vi "Example Write File.vi"() -> ()   [LabVIEW 2013]
uses:
  C:/tf/play/labview/Tinkerforge.dll
  Tinkerforge.dll
panel:
  out "transferred (byte)":i32
  in  "local path":path=path "C:/foobar.txt"
  in  "remote path":string="/home/tf/foobar.txt"
  in  "uid":string="XXYYZZ"
  in  "port":i32=4223
  in  "host":string="localhost"
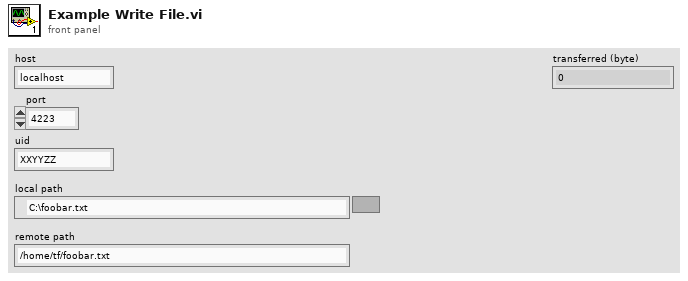
[diagram p1: front panel]
types:
  T1 = enum16{"open", "replace", "create", "open or create", "replace or create", "replace or create with confirmation"}
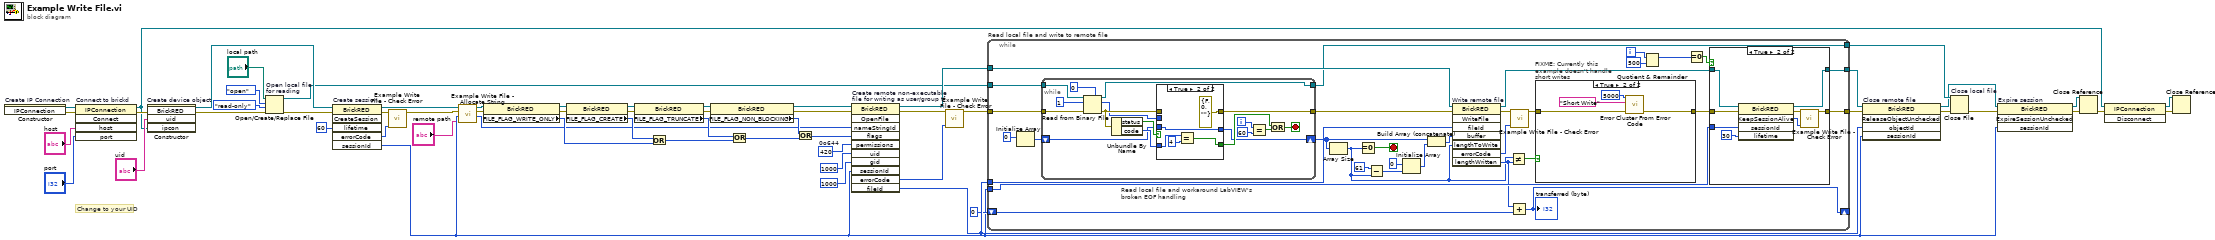
[diagram p0: block diagram]
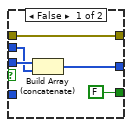
[diagram p2: hidden frame]
diagram:
  w41 = 420  # 0o644
  # "Change to your UID"
  n1 = constructor on="Create IP Connection" class="IPConnection"() -> (reference out=w59:refnum<k24>, error out=w49:errorcluster)  [unwired: 3 in, 1 out]
  n2 = invoke on="Connect to brickd" class="IPConnection" method="Connect"(reference=w59, error in=w49, "host"="host", "port"="port") -> (reference out=w51:refnum<k24>, error out=w55:errorcluster)  [unwired: 1 in, 3 out]
  n3 = constructor on="Create device object" class="BrickRED"(error in=w55, "uid"="uid", "ipcon"=w51) -> (reference out=w54:refnum<k24>, error out=w25:errorcluster)  [unwired: 2 in, 3 out]
  n4 = Open/Create/Replace File "Open local file\nfor reading"(file path (use dialog)="local path", error in=w25, operation (0:open)=T1."open", access (0:read/write)=enum16{"read/write", "read-only", "write-only"}."read-only") -> (refnum out=w35:refnum<file>, error out=w24:errorcluster)  [unwired: 2 in, 1 out]
  n5 = invoke on="Create session" class="BrickRED" method="CreateSession"(reference=w54, error in=w24, "lifetime"=i64 60) -> (reference out=w6:refnum<k24>, error out=w47:errorcluster, "errorCode"=w46:u8, "sessionId"=w2:i32)  [unwired: 3 in, 2 out]
  n6 = call "Example Write File - Check Error.vi"("error code"=w46, "error in"=w47) -> ("error out"=w7:errorcluster)  [unwired: 9 in]
  n7 = call "Example Write File - Allocate String.vi"("buffer"="remote path", "session id"=w2, "error in"=w7, "reference in"=w6) -> ("string id"=w3:i32, "error out"=w4:errorcluster, "reference out"=w5:refnum<k24>)  [unwired: 5 in]
  n8 = property class="BrickRED"(reference=w5, error in=w4) -> (reference out=w22:refnum<k24>, error out=w23:errorcluster, "FILE_FLAG_WRITE_ONLY"=w20:i64)
  n9 = property class="BrickRED"(reference=w22, error in=w23) -> (reference out=w18:refnum<k24>, error out=w15:errorcluster, "FILE_FLAG_CREATE"=w21:i64)
  n10 = property class="BrickRED"(reference=w18, error in=w15) -> (reference out=w17:refnum<k24>, error out=w16:errorcluster, "FILE_FLAG_TRUNCATE"=w14:i64)
  n11 = Or(x=w21, y=w20) -> (x .or. y?=w19:i64)
  n12 = property class="BrickRED"(reference=w17, error in=w16) -> (reference out=w39:refnum<k24>, error out=w40:errorcluster, "FILE_FLAG_NON_BLOCKING"=w11:i64)
  n13 = Or(x=w14, y=w19) -> (x .or. y?=w12:i64)
  n14 = Or(x=w11, y=w12) -> (x .or. y?=w13:i64)
  n15 = invoke on="Create remote non-executable\nfile for writing as user/group tf" class="BrickRED" method="OpenFile"(reference=w39, error in=w40, "nameStringId"=w3, "flags"=w13, "permissions"=w41, "uid"=i64 1000, "gid"=i64 1000, "sessionId"=w2) -> (reference out=w36:refnum<k24>, error out=w44:errorcluster, "errorCode"=w45:u8, "fileId"=w33:i32)  [unwired: 3 in, 7 out]
  n16 = call "Example Write File - Check Error.vi"("error code"=w45, "error in"=w44) -> ("error out"=w26:errorcluster)  [unwired: 9 in]
  n17 = while "Read local file and write to remote file" {
    tunnel: w26 -> [w73]
    tunnel: [w82] -> w10
    tunnel: w36 -> [w91]
    tunnel: [w83] -> w32
    tunnel: w33 -> [w90]
    tunnel: w35 -> [w71]
    tunnel: [w70] -> w34
    tunnel: w2 -> [w81]
    shift-right: [w80] -> _
    shift-left: 0 -> [w79]
    i -> [w88]
    stop <- w60 stop-if-true
    n18 = Initialize Array(u8 0) -> (w68:u8[])  [unwired: 1 in]
    n19 = while "Read local file and workaround LabVIEW's broken EOF handling" {
      tunnel: w73 -> [w108]
      tunnel: [w104] -> w72
      tunnel: w71 -> [w107]
      tunnel: [w106] -> w70
      shift-right: [w93] -> w64
      shift-left: w68 -> [w92]
      i -> [w98]
      stop <- w99 stop-if-true
      n20 = Read from Binary File(5:u8 0, 8:w108, 10:1 ("count (1)"), 11:w107) -> (0:w103:errorcluster, 2:w94:u8[], 3:w106:refnum<file>)  [unwired: 2 in, 1 out]
      n21 = Unbundle By Name(w103) -> ("status"=w96:bool, "code"=w102:i32)
      n22 = case shown="True" w96 {
        tunnel: [w113 errorcluster {"status"=FALSE, "code"=0, "source"=""} ("error out")] -> w104
        tunnel: w103 -> [w113 _]
        tunnel: w102 -> [_ w118]
        tunnel: [FALSE w116] -> w100
        tunnel: w94 -> [w109 _]
        tunnel: [w111 w114] -> w93
        tunnel: w92 -> [w110 w114]
        frame False {
          n23 = Build Array (concatenate)(w110, w109) -> (w111:u8[])
        }
        frame True {
          n24 = Equal?(x=w118, y=4) -> (x = y?=w116:bool)
        }
      }
      n25 = Equal?(x=w98, y=60) -> (x = y?=w101:bool)
      n26 = Or(x=w100, y=w101) -> (x .or. y?=w99:bool)
    }
    n27 = Array Size(array=w64) -> (size(s)=w61:i32)
    n28 = Equal To 0?(x=w61) -> (x = 0?=w60:bool)
    n29 = Subtract(x=61, y=w61) -> (x-y=w65:i32)
    n30 = Initialize Array(u8 0, w65) -> (w63:u8[])
    n31 = Build Array (concatenate)(w64, w63) -> (w62:u8[])
    n32 = invoke on="Write remote file" class="BrickRED" method="WriteFile"(reference=w91, error in=w72, "fileId"=w90, "buffer"=w62, "lengthToWrite"=w61) -> (reference out=w84:refnum<k24>, error out=w89:errorcluster, "errorCode"=w78:u8, "lengthWritten"=w77:u8)  [unwired: 3 in, 4 out]
    n33 = Not Equal?(x=w61, y=w77) -> (x != y?=w76:bool)
    n34 = Add(x=w77, y=w79) -> (x+y=w80:i32)
    "transferred (byte)" <- w80
    n35 = call "Example Write File - Check Error.vi"("error code"=w78, "error in"=w89) -> ("error out"=w75:errorcluster)  [unwired: 9 in]
    n36 = case "FIXME: Currently this example doesn't handle short writes" shown="True" w76 {
      tunnel: w75 -> [w119 w123]
      tunnel: [w119 w122] -> w74
      frame False {
      }
      frame True {
        n37 = call <vilib>:"Error Cluster From Error Code.vi"("error in (no error)"=w123, "error message (\"\")"="Short Write" ("error message (\"\")"), "error code (0)"=5000) -> ("error out"=w122:errorcluster)  [unwired: 6 in]
      }
    }
    n38 = Quotient & Remainder(x=w88, y=500) -> (x-y*floor(x/y)=w86:i32)  [unwired: 1 out]
    n39 = Equal To 0?(x=w86) -> (x = 0?=w85:bool)
    n40 = case shown="True" w85 {
      tunnel: w84 -> [w125 w133]
      tunnel: [w125 w132] -> w83
      tunnel: w74 -> [w124 w131]
      tunnel: [w124 w126] -> w82
      tunnel: w81 -> [_ w130]
      frame False {
      }
      frame True {
        n41 = invoke class="BrickRED" method="KeepSessionAlive"(reference=w133, error in=w131, "sessionId"=w130, "lifetime"=i64 30) -> (reference out=w132:refnum<k24>, error out=w127:errorcluster, "KeepSessionAlive"=w128:u8)  [unwired: 1 in, 2 out]
        n42 = call "Example Write File - Check Error.vi"("error code"=w128, "error in"=w127) -> ("error out"=w126:errorcluster)  [unwired: 9 in]
      }
    }
  }
  n43 = invoke on="Close remote file" class="BrickRED" method="ReleaseObjectUnchecked"(reference=w32, error in=w10, "objectId"=w33, "sessionId"=w2) -> (reference out=w31:refnum<k24>, error out=w9:errorcluster)  [unwired: 1 in, 3 out]
  n44 = Close File "Close local file"(refnum=w34, error in=w9) -> (error out=w8:errorcluster)  [unwired: 1 out]
  n45 = invoke on="Expire session" class="BrickRED" method="ExpireSessionUnchecked"(reference=w31, error in=w8, "sessionId"=w2) -> (reference out=w30:refnum<k24>, error out=w29:errorcluster)  [unwired: 1 in, 2 out]
  n46 = Close Reference(reference=w30, error in (no error)=w29) -> (error out=w53:errorcluster)
  n47 = invoke class="IPConnection" method="Disconnect"(reference=w51, error in=w53) -> (reference out=w50:refnum<k24>, error out=w52:errorcluster)  [unwired: 1 in, 1 out]
  n48 = Close Reference(reference=w50, error in (no error)=w52) -> ()  [unwired: 1 out]
